vi "Required Buffer Size (Transfer Group).vi"(8 "error in (no error)":errorcluster, 9 "initial engine buffer size (0)":u64 format="%d bytes", 10 "initial string buffer size (0)":u64 format="%d bytes", 11 "Transfer Group Configuration in":T1={"name"="", "direction"=enum."Tx", "cycle timing"={"priority"=0, "decimation"=1, "offset"=0}, "thread index"=-1, "settings"=[], "Transfers"=[], "timeout behavior"=enum."Increment Late Count"} {"Transfers"."channels"."string offset" format="%d bytes"}) -> (0 "error out":errorcluster, 1 "total engine buffer size":u64 format="%d bytes", 2 "total string buffer size":u64 format="%d bytes", 3 "Transfer Group Configuration out":T1={"name"="", "direction"=enum."Tx", "cycle timing"={"priority"=0, "decimation"=1, "offset"=0}, "thread index"=-1, "settings"=[], "Transfers"=[], "timeout behavior"=enum."Increment Late Count"} {"Transfers"."channels"."string offset" format="%d bytes"})   [LabVIEW 2017, in "DSF Core.lvlib"]
uses:
  DSF Core.lvlib
  Typedefs/DSF Engine Transfer Group Configuration.ctl
  Typedefs/DSF Direction.ctl
  Typedefs/DSF Timing Info.ctl
  Typedefs/DSF Settings Info.ctl
  Typedefs/DSF Engine Transfer Configuration.ctl
  Typedefs/DSF Byte Order.ctl
  Typedefs/DSF Engine Channel Configuration.ctl
  Typedefs/DSF Data Type.ctl
  Typedefs/DSF Timeout Behavior.ctl
  VIs/Sizeof.vi
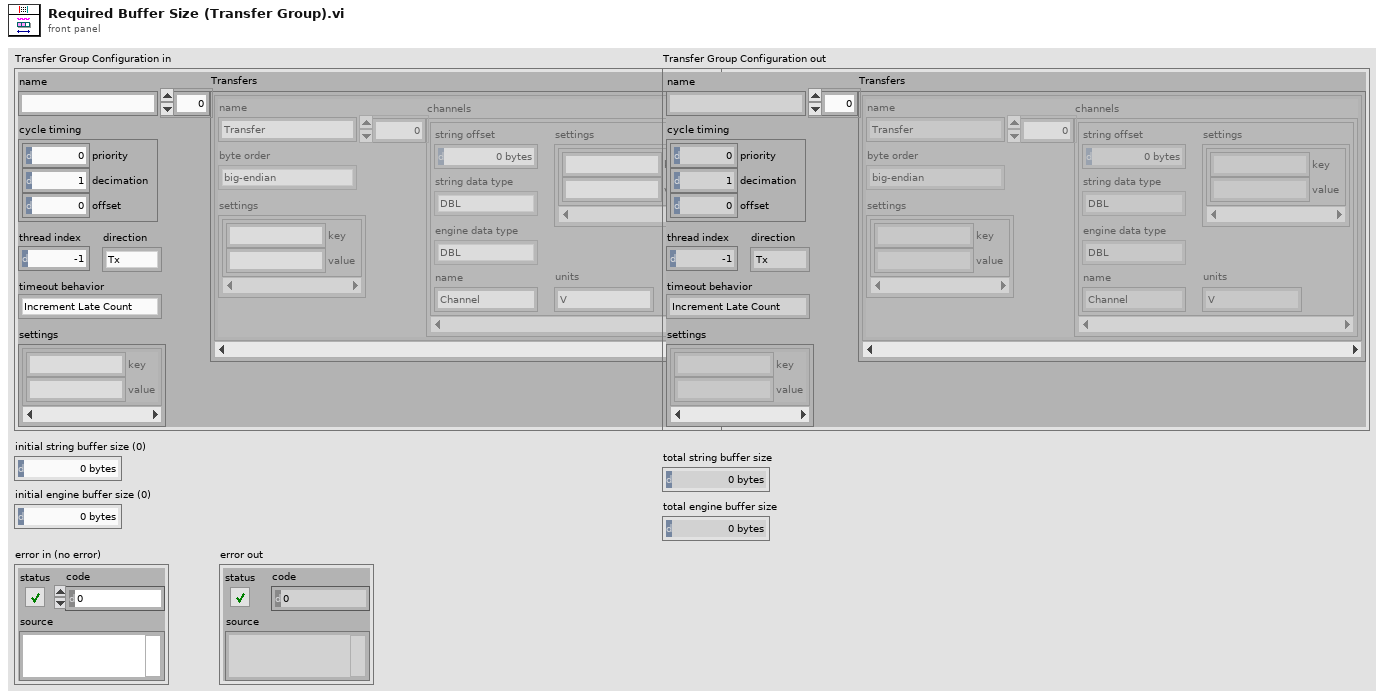
[diagram p1: front panel]
types:
  T1 = typedef "DSF Core.lvlib/DSF Engine Transfer Group Configuration.ctl" = cluster{"name":string, "direction":T2, "cycle timing":T3, "thread index":i32, "settings":T4, "Transfers":T5[], "timeout behavior":T9}
  T2 = typedef "DSF Core.lvlib/DSF Direction.ctl" = enum8{"Tx", "Rx"}
  T3 = typedef "DSF Core.lvlib/DSF Timing Info.ctl" = cluster{"priority":u64, "decimation":u64, "offset":u64}
  T4 = typedef "DSF Core.lvlib/DSF Settings Info.ctl" = cluster{"key":string, "value":string}[]
  T5 = typedef "DSF Core.lvlib/DSF Engine Transfer Configuration.ctl" = cluster{"name":string, "byte order":T6, "settings":T4, "channels":T7[]}
  T6 = typedef "DSF Core.lvlib/DSF Byte Order.ctl" = enum8{"big-endian", "little-endian"}
  T7 = typedef "DSF Core.lvlib/DSF Engine Channel Configuration.ctl" = cluster{"string offset":u64, "string data type":T8, "engine data type":T8, "name":string, "settings":T4, "units":string}
  T8 = typedef "DSF Core.lvlib/DSF Data Type.ctl" = enum8{"Bool", "SGL", "DBL", "I8", "I16", "I32", "I64", "U8", "U16", "U32", "U64"}
  T9 = typedef "DSF Core.lvlib/DSF Timeout Behavior.ctl" = enum8{"Increment Late Count", "Throw Error"}
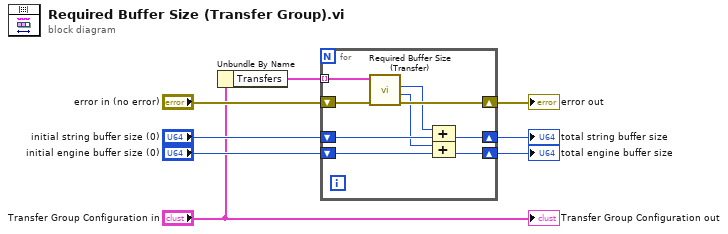
[diagram p0: block diagram]
diagram:
  n1 = Unbundle By Name("Transfer Group Configuration in") -> ("Transfers"=w7:T5[])
  n2 = for {
    tunnel: w7 -> [w17] mode=indexing
    shift-right: [w10] -> w8
    shift-left: "initial string buffer size (0)" -> [w14]
    shift-right: [w16] -> w5
    shift-left: "error in (no error)" -> [w15]
    shift-right: [w11] -> w4
    shift-left: "initial engine buffer size (0)" -> [w12]
    n3 = call "Required Buffer Size (Transfer).vi"("error in (no error)"=w15, "Transfer Configuration in"=w17) -> ("error out"=w16:errorcluster, "engine buffer size"=w13:u64, "string buffer size"=w9:u64)  [unwired: 6 in, 1 out]
    n4 = Compound Arithmetic op=ADD(w9, w14) -> (w10:u64)
    n5 = Compound Arithmetic op=ADD(w13, w12) -> (w11:u64)
  }
  "total string buffer size" <- w8
  "error out" <- w5
  "total engine buffer size" <- w4
  "Transfer Group Configuration out" <- "Transfer Group Configuration in"
